vi "Update Alliance State.vi"   [LabVIEW 2016]
uses:
  Robot Values.vi
  Robot Global Data.vi
  <vilib>/Rock Robotics/WPI/DriverStation/WPI_DriverStationRobotMode2.ctl
  <vilib>/Rock Robotics/WPI/DriverStation/WPI_DriverStationAllianceInfo.ctl
  LED Send Global.vi
types:
  T1 = typedef "WPI_DriverStationAllianceInfo.ctl" = enum16{"Red", "Blue", "Invalid"}
  T2 = typedef "WPI_DriverStationRobotMode2.ctl" = enum16{"Autonomous Disabled", "Autonomous Enabled", "Teleop Disabled", "Teleop Enabled", "Disconnected", "Finish", "Test Disabled", "Test Enabled", "Emergency Stopped"}
  T3 = typedef "WPI_DriverStationPositionInfo.ctl" = enum16{"1", "2", "3"}
  T4 = typedef "LED Send Global.ctl" = cluster{"Underglow States":cluster{"RED":bool, "BLUE":bool}, "Hopper States":cluster{"No Shooter Power":bool, "1 RED":bool, "2 RED":bool, "3 RED":bool, "1 YEL 3 RED":bool, "2 YEL 3 RED":bool, "3 YEL 3 RED":bool, "1 GRN 3 YEL 3 RED":bool, "2 GRN 3 YEL 3 RED":bool, "3 GRN 3 YEL 3 RED":bool, "All GRN":bool, "Shooter w/Agitator":bool}, "License Plate States":cluster{"Auton States":cluster{"Do Nothing":bool, "Gear":bool, "Gear & Baseline":bool, "Gear & Shooter":bool, "Shooter":bool, "Shooter & Ball Dump":bool}, "Drive Train":cluster{"High Gear":bool, "Low Gear":bool}}, "Misc":cluster{"Pit/Demo":bool}, "Lights":cluster{"Underglow":string, "License Plate":string, "Hopper":string}}
  T5 = typedef "Robot Values.ctl" = cluster{"Robot Drive":cluster{"Left Motor Power":dbl, "Right Motor Power":dbl, "Left Encoder Value":dbl, "Right Encoder Value":dbl, "High Gear?":bool, "PTO?":bool}, "Sensors":cluster{"Gyro Angle":u16, "Recalibrate Gyro":bool, "Reset Gyro":bool}, "Shooter":cluster{"Prep Wheels":bool, "Shoot":bool, "Left Shooter Wheel Speed":dbl, "Wheels Moving":bool, "Shooter Prepped":bool, "Shooter RPS SP":dbl, "Shooting?":bool, "Left Shooter Wheel Power":dbl, "Right Shooter Wheel Power":dbl, "Acquisition Conveyor Power":dbl, "Hopper Beater Bar Power":dbl, "Filtered Left Shooter Speed":dbl, "Acquisition Motor Power":dbl, "Joystick Add":dbl}, "Robot States":cluster{"Drive mode":string, "Alliance":T1, "Position":T3}, "Gear":cluster{"Ejection Active":bool}, "Lights":cluster{"Underglow":string, "License Plate":string, "Hopper":string}}
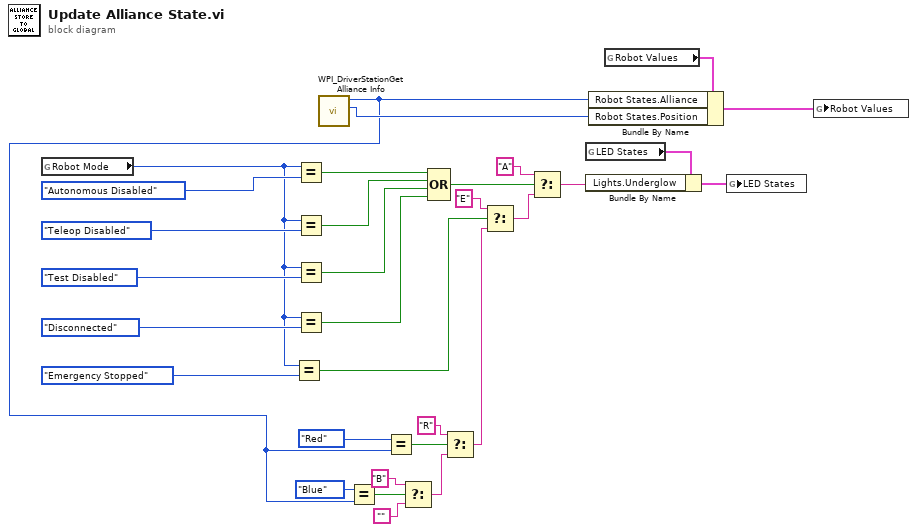
[diagram p0: block diagram]
diagram:
  n1 = global read "Robot Global Data.vi" "Robot Mode"() -> (w17:T2)
  n2 = Equal?(x=w17, y=WPI_DriverStationRobotMode2."Emergency Stopped" ("Robot Mode")) -> (x = y?=w14:bool)
  n3 = Equal?(x=w17, y=WPI_DriverStationRobotMode2."Autonomous Disabled" ("Robot Mode")) -> (x = y?=w26:bool)
  n4 = Equal?(x=w17, y=WPI_DriverStationRobotMode2."Teleop Disabled" ("Robot Mode")) -> (x = y?=w24:bool)
  n5 = Equal?(x=w17, y=WPI_DriverStationRobotMode2."Test Disabled" ("Robot Mode")) -> (x = y?=w21:bool)
  n6 = Equal?(x=w17, y=WPI_DriverStationRobotMode2."Disconnected" ("Robot Mode")) -> (x = y?=w20:bool)
  n7 = call <vilib>:"WPI_DriverStationGet Alliance Info.vi"() -> ("Position"=w29:T3, "Alliance"=w28:T1)  [unwired: 10 in]
  n8 = Equal?(x=WPI_DriverStationAllianceInfo."Blue" ("Alliance"), y=w28) -> (x = y?=w6:bool)
  n9 = Equal?(x=WPI_DriverStationAllianceInfo."Red" ("Alliance"), y=w28) -> (x = y?=w10:bool)
  n10 = Select(t="B", s=w6, f="") -> (s? t:f=w9:string)
  n11 = Compound Arithmetic op=OR(w26, w24, w21, w20) -> (w19:bool)
  n12 = Select(t="R", s=w10, f=w9) -> (s? t:f=w5:string)
  n13 = Select(t="E", s=w14, f=w5) -> (s? t:f=w15:string)
  n14 = Select(t="A", s=w19, f=w15) -> (s? t:f=w3:string)
  n15 = global read "LED Send Global.vi" "LED States"() -> (w2:T4)
  n16 = Bundle By Name(cluster=w2, "Lights.Underglow"=w3) -> (w1:T4)
  n17 = global read "Robot Values.vi" "Robot Values"() -> (w31:T5)
  n18 = Bundle By Name(cluster=w31, "Robot States.Alliance"=w28, "Robot States.Position"=w29) -> (w30:T5)
  n19 = global write "LED Send Global.vi" "LED States"(w1) -> ()
  n20 = global write "Robot Values.vi" "Robot Values"(w30) -> ()
